vi "Write ActorMap-Models.vi"(8 "error in (no error)":errorcluster, 10 "ActorMap.lvclass":refnum<class "ActorMap.lvclass">, 11 "MVVM Abstruct Controller in":refnum<class "MVVM Abstruct Controller.lvclass">) -> (0 "error out":errorcluster, 3 "MVVM Abstruct Controller out":refnum<class "MVVM Abstruct Controller.lvclass">)   [LabVIEW 2020, in "MMVVM Framework.lvlib" / "MVVM Abstruct Controller.lvlib" / "MVVM Abstruct Controller.lvclass"]
uses:
  MVVM Abstruct Controller.lvclass
  ActorMap/ActorMap.lvclass
  MVVM Abstruct Controller.lvclass/MVVM Abstruct Controller.ctl
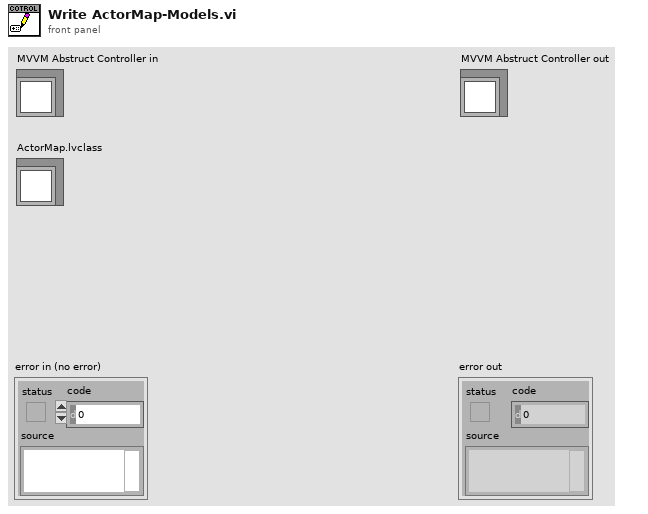
[diagram p1: front panel]
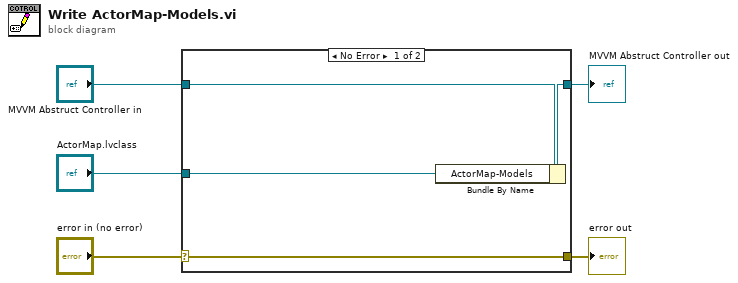
[diagram p0: block diagram]
diagram:
  n1 = case shown="No Error" "error in (no error)" {
    selector: "error in (no error)" -> [w9 w10]
    tunnel: [w9 w10] -> w4
    tunnel: [w7 w11] -> w2
    tunnel: "MVVM Abstruct Controller in" -> [w8 w11]
    tunnel: "ActorMap.lvclass" -> [w6 _]
    frame No Error {
      n2 = Bundle By Name(cluster=w8, "ActorMap-Models"=w6) -> (w7:refnum<class "MVVM Abstruct Controller.lvclass">)
    }
    frame Error {
    }
  }
  "error out" <- w4
  "MVVM Abstruct Controller out" <- w2
